vi "FPGA_DIOReadDI.vi"(8 "error in (no error)":errorcluster, 11 "DIODeviceRef":T1) -> (0 "error out":errorcluster, 2 "DI":u32, 3 "DIODeviceRef":T1)   [LabVIEW 2017]
uses:
  <vilib>/Rock Robotics/SystemInterfaces/DIO/FPGA_DIODevRef.ctl
  <vilib>/Rock Robotics/SystemInterfaces/System/FPGA_SystemFPGA Ref Global.vi
  <vilib>/Utility/error.llb/Error Cluster From Error Code.vi
  <vilib>/rvi/errors/niLvFpgaAdjustHostInterfaceError.vi
  <vilib>/rvi/interface/nirviReadWriteControl/nirviReadWriteControl.xnode
  <vilib>/Rock Robotics/SystemInterfaces/System/FPGA_SystemFRC FPGA Ref.ctl
  NiFpgaLv.dll
  <vilib>/rvi/interface/Simulation/niFpgaSimulationCallBeginRW.vi
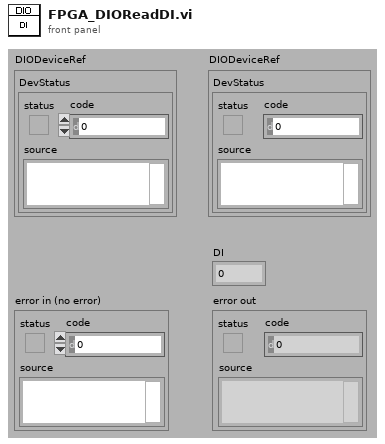
[diagram p1: front panel]
types:
  T1 = typedef "FPGA_DIODevRef.ctl" = cluster{"DevStatus":errorcluster}
  T2 = typedef "FPGA_SystemFRC FPGA Ref.ctl" = refnum<k20>
  T3 = cluster{"Headers":fxp<+,10,10>, "SPIPort":fxp<+,5,5>, "Reserved":fxp<+,1,1>, "MXP":u16}
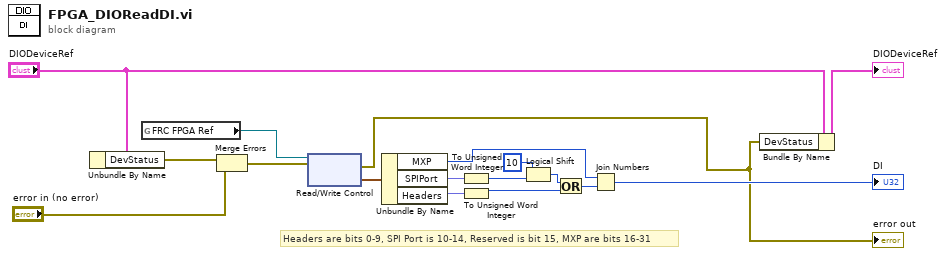
[diagram p0: block diagram]
diagram:
  # "Headers are bits 0-9, SPI Port is 10-14, Reserved is bit 15, MXP are bits 16-31"
  n1 = Unbundle By Name("DIODeviceRef") -> ("DevStatus"=w13:errorcluster)
  n2 = global read "FPGA_SystemFPGA Ref Global.vi" "FRC FPGA Ref"() -> (w14:T2)
  n3 = Merge Errors(w13, "error in (no error)") -> (w12:errorcluster)
  n4 = xnode "Read/Write Control"("FPGA VI Reference In"=w14, "error in"=w12) -> ("error out"=w11:errorcluster, "DIO.DI"=w10:T3)  [unwired: 1 out]
  "error out" <- w11
  n5 = Unbundle By Name(w10) -> ("MXP"=w6:u16, "SPIPort"=w7:fxp<+,5,5>, "Headers"=w8:fxp<+,10,10>)
  n6 = To Unsigned Word Integer(number=w7) -> (unsigned 16bit integer=w4:u16)
  n7 = To Unsigned Word Integer(number=w8) -> (unsigned 16bit integer=w1:u16)
  n8 = Logical Shift(y=i16 10, x=w4) -> (x << y=w2:u16)
  n9 = Or(x=w2, y=w1) -> (x .or. y?=w3:u16)
  n10 = Join Numbers(hi=w6, lo=w3) -> ((hi.lo)=→"DI":u32)
  n11 = Bundle By Name(cluster="DIODeviceRef", "DevStatus"=w11) -> (→"DIODeviceRef":T1)
